vi "test Add-Find-Remove Subaddress.vi"(8 "error in":errorcluster, 11 "TestCase in":refnum<class "Scripting.lvclass">) -> (0 "error out":errorcluster, 3 "TestCase out":refnum<class "Scripting.lvclass">)   [LabVIEW 2020, in "Scripting.lvclass"]
uses:
  Scripting.lvclass
  <vilib>/addons/_JKI Toolkits/VI Tester/TestCase.llb/TestCase.lvclass
  Scripting/Ballard MIL-STD-1553 Scripting.lvlib
  <vilib>/NI VeriStand/Custom Device API/Custom Device Item Ref.ctl
  <vilib>/NI VeriStand/Custom Device API/Custom Device API.lvlib
  Shared/Address.ctl
  C:/Program Files (x86)/National Instruments/LabVIEW 2020/vi.lib/addons/_JKI Toolkits/VI Tester/TestCase.llb/TestCase.lvclass
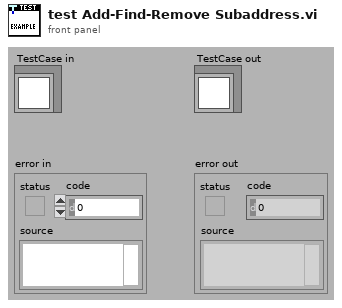
[diagram p1: front panel]
types:
  T1 = typedef "Address.ctl" = u16
  T2 = typedef "Custom Device API.lvlib/Custom Device Item Ref.ctl" = u64
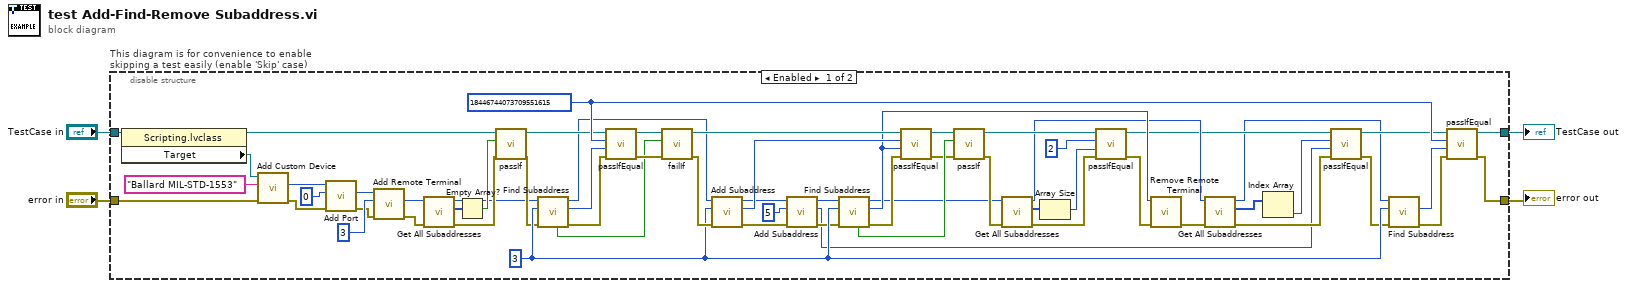
[diagram p0: block diagram]
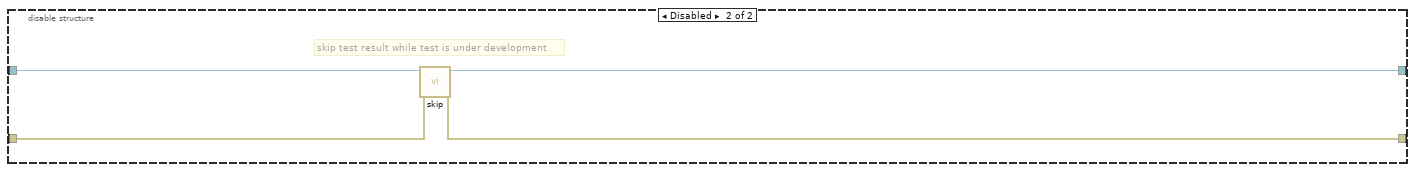
[diagram p2: hidden frame]
diagram:
  n1 = disable-structure "This diagram is for convenience to enable skipping a test easily (enable 'Skip' case)" shown="Enabled" {
    disable-tunnel: "TestCase in" -> [w64 w70]
    disable-tunnel: [w59 w68] -> w1
    disable-tunnel: [w60 w69] -> w3
    disable-tunnel: "error in" -> [w66 w67]
    frame Enabled {
      w44 = T1 3 ("terminal address")
      w49 = T2 18446744073709551615 ("bus controller")
      n2 = property class="Scripting.lvclass"(reference=w64) -> (reference out=w41:refnum<class "Scripting.lvclass">, "Target"=w63:refnum<k24>)  [unwired: 1 in, 1 out]
      n3 = call "Add Custom Device.vi"("error in"=w66, "name"="Ballard MIL-STD-1553", "target in"=w63) -> ("error out"=w38:errorcluster, "Ballard MIL-STD 1553 custom device"=w39:T2)  [unwired: 6 in, 1 out]
      n4 = call "Add Port.vi"("error in"=w38, "port number"=u16 0, "Ballard MIL-STD 1553 custom device in"=w39) -> ("error out"=w8:errorcluster, "port"=w10:T2)  [unwired: 6 in, 1 out]
      n5 = call "Add Remote Terminal.vi"("error in"=w8, "terminal address"=T1 3, "port in"=w10) -> ("error out"=w7:errorcluster, "remote terminal"=w6:T2)  [unwired: 6 in, 1 out]
      n6 = call "Get All Subaddresses.vi"("error in"=w7, "remote terminal in"=w6) -> ("error out"=w37:errorcluster, "subaddresses"=w42:T2[], "remote terminal out"=w35:T2)  [unwired: 7 in]
      n7 = Empty Array?(array=w42) -> (empty?=w43:bool)
      n8 = call-dynamic "passIf.vi"("error in (no error)"=w37, "pass"=w43, "TestCase in"=w41) -> ("error out"=w36:errorcluster, "TestCase out"=w40:refnum<class "Scripting.lvclass">)  [unwired: 7 in]
      n9 = call "Find Subaddress.vi"("error in"=w36, "subaddress value"=w44, "remote terminal in"=w35) -> ("error out"=w57:errorcluster, "subaddress"=w55:T2, "remote terminal out"=w18:T2, "found?"=w45:bool)  [unwired: 5 in]
      n10 = call-dynamic "passIfEqual.vi"("error in (no error)"=w57, "y"=w55, "x"=w49, "TestCase in"=w40) -> ("error out"=w56:errorcluster, "TestCase out"=w46:refnum<class "Scripting.lvclass">)  [unwired: 6 in]
      n11 = call-dynamic "failIf.vi"("error in (no error)"=w56, "fail"=w45, "TestCase in"=w46) -> ("error out"=w58:errorcluster, "TestCase out"=w54:refnum<class "Scripting.lvclass">)  [unwired: 7 in]
      n12 = call "Add Subaddress.vi"("error in"=w58, "subaddress"=w44, "remote terminal in"=w18) -> ("error out"=w31:errorcluster, "subaddress ref"=w53:T2, "remote terminal in"=w32:T2)  [unwired: 6 in]
      n13 = call "Add Subaddress.vi"("error in"=w31, "subaddress"=T1 5 ("terminal address"), "remote terminal in"=w32) -> ("error out"=w34:errorcluster, "subaddress ref"=w11:T2, "remote terminal in"=w33:T2)  [unwired: 6 in]
      n14 = call "Find Subaddress.vi"("error in"=w34, "subaddress value"=w44, "remote terminal in"=w33) -> ("error out"=w52:errorcluster, "subaddress"=w28:T2, "remote terminal out"=w27:T2, "found?"=w51:bool)  [unwired: 5 in]
      n15 = call-dynamic "passIfEqual.vi"("error in (no error)"=w52, "y"=w28, "x"=w53, "TestCase in"=w54) -> ("error out"=w50:errorcluster, "TestCase out"=w61:refnum<class "Scripting.lvclass">)  [unwired: 6 in]
      n16 = call-dynamic "passIf.vi"("error in (no error)"=w50, "pass"=w51, "TestCase in"=w61) -> ("error out"=w29:errorcluster, "TestCase out"=w26:refnum<class "Scripting.lvclass">)  [unwired: 7 in]
      n17 = call "Get All Subaddresses.vi"("error in"=w29, "remote terminal in"=w27) -> ("error out"=w25:errorcluster, "subaddresses"=w24:T2[], "remote terminal out"=w19:T2)  [unwired: 7 in]
      n18 = Array Size(array=w24) -> (size(s)=w23:i32)
      n19 = call-dynamic "passIfEqual.vi"("error in (no error)"=w25, "y"=w23, "x"=2 ("size(s)"), "TestCase in"=w26) -> ("error out"=w21:errorcluster, "TestCase out"=w16:refnum<class "Scripting.lvclass">)  [unwired: 6 in]
      n20 = call "Remove Remote Terminal.vi"("error in"=w21, "remote terminal"=w28) -> ("error out"=w20:errorcluster)  [unwired: 9 in]
      n21 = call "Get All Subaddresses.vi"("error in"=w20, "remote terminal in"=w19) -> ("error out"=w14:errorcluster, "subaddresses"=w17:T2[], "remote terminal out"=w12:T2)  [unwired: 7 in]
      n22 = Index Array(array=w17) -> (element=w5:T2)  [unwired: 1 in]
      n23 = call-dynamic "passIfEqual.vi"("error in (no error)"=w14, "y"=w11, "x"=w5, "TestCase in"=w16) -> ("error out"=w13:errorcluster, "TestCase out"=w15:refnum<class "Scripting.lvclass">)  [unwired: 6 in]
      n24 = call "Find Subaddress.vi"("error in"=w13, "subaddress value"=w44, "remote terminal in"=w12) -> ("error out"=w47:errorcluster, "subaddress"=w48:T2)  [unwired: 5 in, 2 out]
      n25 = call-dynamic "passIfEqual.vi"("error in (no error)"=w47, "y"=w48, "x"=w49, "TestCase in"=w15) -> ("error out"=w60:errorcluster, "TestCase out"=w59:refnum<class "Scripting.lvclass">)  [unwired: 6 in]
    }
    frame Disabled {
      # "skip test result while test is under development"
      n26 = call <vilib>:"skip.vi"("error in (no error)"=w67, "TestCase in"=w70) -> ("error out"=w69:errorcluster, "TestCase out"=w68:refnum<class "Scripting.lvclass">)  [unwired: 8 in]
    }
  }
  "error out" <- w3
  "TestCase out" <- w1
